vi "Write Text_Header.vi"(8 "error in (no error)":errorcluster caption="에러 입력(에러 없음)", 10 "Text_Header":u16[](array[numeric]) format="%x", 11 "Text File 입력":refnum<class "Text File.lvclass">) -> (0 "error out":errorcluster caption="에러 출력", 3 "Text File 출력":refnum<class "Text File.lvclass">)   [LabVIEW 2020, in "Text File.lvclass"]
uses:
  Text File.lvclass
  Text File.lvclass/Text File.ctl
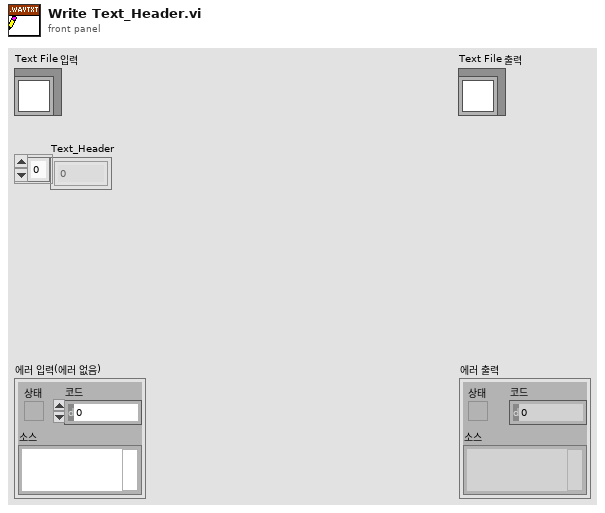
[diagram p1: front panel]
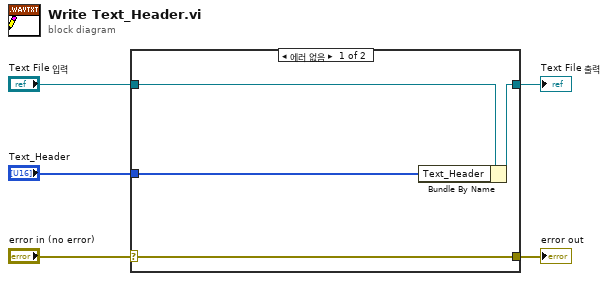
[diagram p0: block diagram]
diagram:
  n1 = case shown="에러 없음" "error in (no error)" {
    selector: "error in (no error)" -> [w9 w10]
    tunnel: [w9 w10] -> w4
    tunnel: [w7 w11] -> w2
    tunnel: "Text File 입력" -> [w8 w11]
    tunnel: "Text_Header" -> [w6 _]
    frame No Error {
      n2 = Bundle By Name(cluster=w8, "Text_Header"=w6) -> (w7:refnum<class "Text File.lvclass">)
    }
    frame Error {
    }
  }
  "error out" <- w4
  "Text File 출력" <- w2
